vi "Control Mode Write Array.vi"(8 "error in":errorcluster, 10 "Control Mode STS":u16[](array[numeric]), 11 "Control Mode in":refnum<class "Control Mode.lvclass">) -> (0 "error out":errorcluster, 3 "Control Mode out":refnum<class "Control Mode.lvclass">)   [LabVIEW 2023, in "Control Mode.lvclass"]
uses:
  Control Mode.lvclass
  Control Mode.lvclass/Control Mode.ctl
  <vilib>/ADAS Replay HIL/Channels/Tag Wrapper/Polymorphic/Write Channel (U16).vi
  <vilib>/ADAS Replay HIL/Channels/Tag Wrapper/Polymorphic/Write Channel (U16).vi/cccb8e89-591f-4bb4-9d4e-ae06ba1f5498.vi
  <vilib>/ADAS Replay HIL/Channels/Tag Wrapper/Polymorphic/Write Channel (U16).vi/cccb8e89-591f-4bb4-9d4e-ae06ba1f5498.vi/4bc1c15b-36ab-481f-b8dd-c64075ce723a.vi
  <vilib>/ADAS Replay HIL/Channels/Tag Wrapper/Polymorphic/Write Channel (U16).vi/cccb8e89-591f-4bb4-9d4e-ae06ba1f5498.vi/d83cb72b-7713-41fc-a3d1-682de79cf574.vi
  <vilib>/ADAS Replay HIL/Channels/Tag Wrapper/Tag Wrapper.lvlib
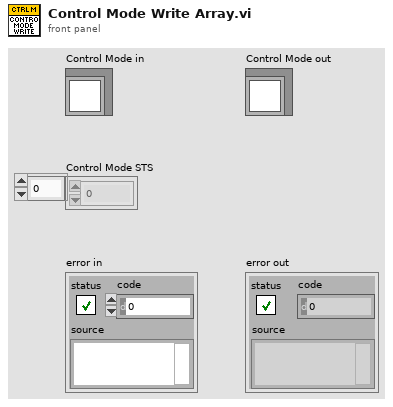
[diagram p1: front panel]
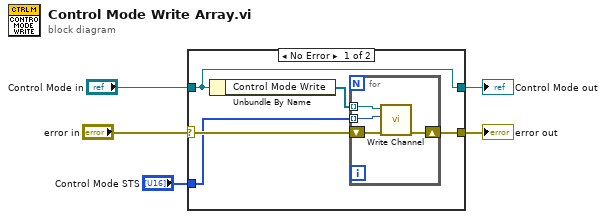
[diagram p0: block diagram]
diagram:
  n1 = case shown="No Error" "error in" {
    selector: "error in" -> [w10 w16]
    tunnel: [w9 w16] -> w3
    tunnel: [w7 w15] -> w4
    tunnel: "Control Mode in" -> [w7 w15]
    tunnel: "Control Mode STS" -> [w6 _]
    frame No Error {
      n2 = Unbundle By Name(w7) -> ("Control Mode Write"=w8:refnum<k21>[])
      n3 = for {
        shift-right: [w13] -> w9
        shift-left: w10 -> [w14]
        tunnel: w8 -> [w12] mode=indexing
        tunnel: w6 -> [w11] mode=indexing
        n4 = call-poly <vilib>:"Write Channel.vi"("error in"=w14, "Value to Write"=w11, "ADAS HIL Channel in"=w12) -> ("error out"=w13:errorcluster)  [unwired: 6 in, 2 out]
      }
    }
    frame Error {
    }
  }
  "error out" <- w3
  "Control Mode out" <- w4
